vi "Configure Channel Characteristics Core.vi"(0 "CS++Scope":refnum<class "CS++Scope.lvclass">, 5 "channel name (\"CHANNEL1\")":string="CHANNEL1", 7 "input impedance (1.0E+6 ohms)":dbl[unit]=1000000.0 format="%.2e", 9 "max input frequency (1.0E+6 Hz)":dbl[unit]=1000000.0 format="%.2e", 11 "error in (no error)":errorcluster) -> (4 "CS++Scope out":refnum<class "CS++Scope.lvclass">, 15 "error out":errorcluster)   [LabVIEW 2014, in "CS++Scope.lvlib" / "CS++Scope.lvclass"]
doc: "This VI configures the properties that control the electrical characteristics of the channel. These properties are the input impedance and the maximum frequency of the input signal."
uses:
  CS++Scope.lvclass
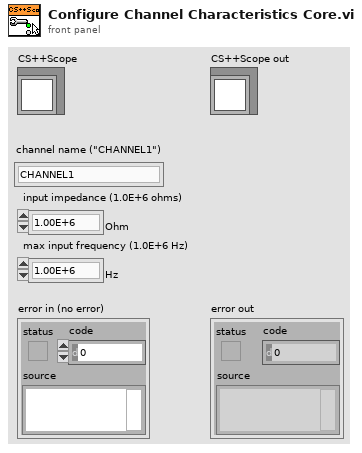
[diagram p1: front panel]
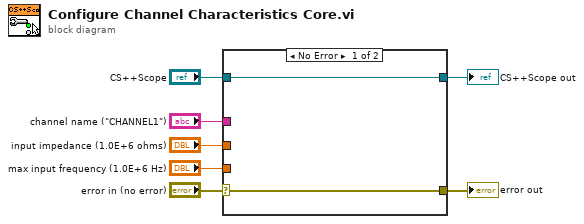
[diagram p0: block diagram]
diagram:
  n1 = case shown="No Error" "error in (no error)" {
    selector: "error in (no error)" -> [w8 w11]
    tunnel: [w8 w11] -> w6
    tunnel: [w9 w10] -> w2
    tunnel: "CS++Scope" -> [w9 w10]
    tunnel: "channel name (\"CHANNEL1\")" -> [_ _]
    tunnel: "input impedance (1.0E+6 ohms)" -> [_ _]
    tunnel: "max input frequency (1.0E+6 Hz)" -> [_ _]
    frame No Error {
    }
    frame Error {
    }
  }
  "error out" <- w6
  "CS++Scope out" <- w2
